vi "map_diag_piastre_stiffback.vi"() -> ()   [LabVIEW 2015]
panel:
  in  "x piastra":bool
  in  "y piastra":bool
  in  "z piastra":bool
  in  "Done":bool
  in  "y inizio":bool
  in  "Positioning Done":bool
  in  "x inizio":bool
  in  "y inizio":bool
  in  "Positioning Done":bool
  in  "y inizio":bool
  in  "Positioning Done":bool
  in  "KILL":bool
  in  "PAUSE":bool
  in  "RESUME":bool
  in  "QUIT":bool
  in  "Positioning Done":bool
  in  "y inizio":bool
  in  "x inizio":bool
  in  "End":bool
  in  "zero z - end":bool
  in  "zero x - end":bool
  in  "zero y - end":bool
  out "output":string
  out "command":string
  in  "zero done":bool
  in  "zero z":bool
  in  "zero x":bool
  in  "zero y":bool
  # "Posiziono in zero"
  # "Comandi di emergenza"
  # "Vado al punto di partenza\nDiagonale Left Internal"
  # "Vado al punto di partenza\nDiagonale Right Internal"
  # "Vado al punto di partenza\nDiagonale Left External"
  # "Vado al punto di partenza\nDiagonale Right External"
  # "Ritorno a zero"
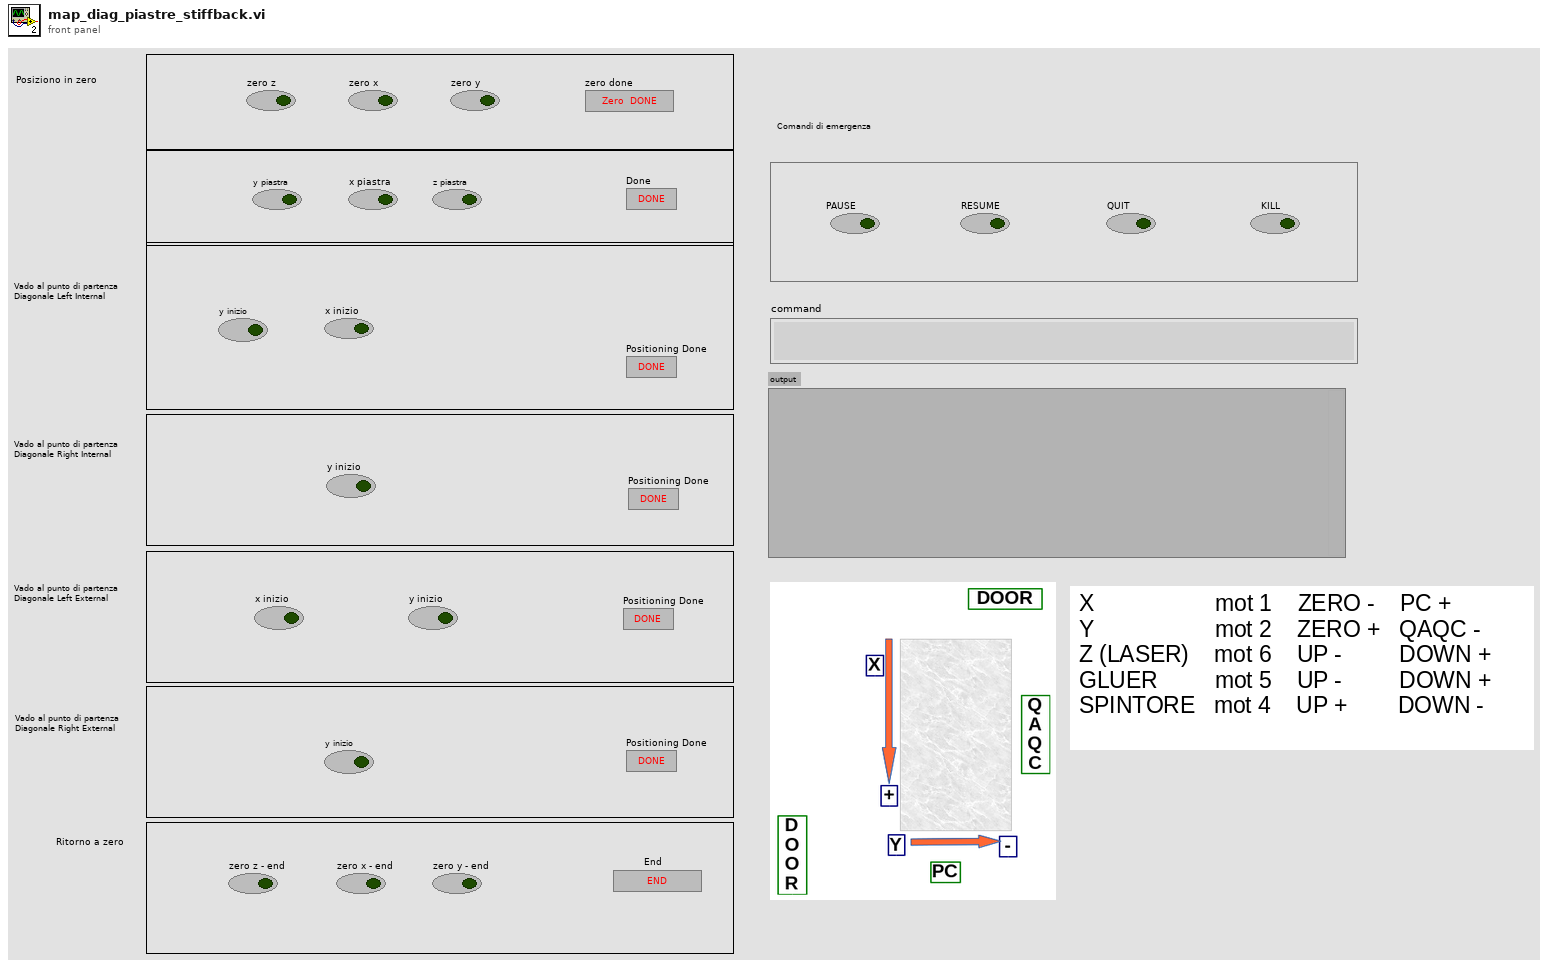
[diagram p1: front panel]
types:
  T1 = enum16{"open", "replace", "create", "open or create", "replace or create", "replace or create with confirmation"}
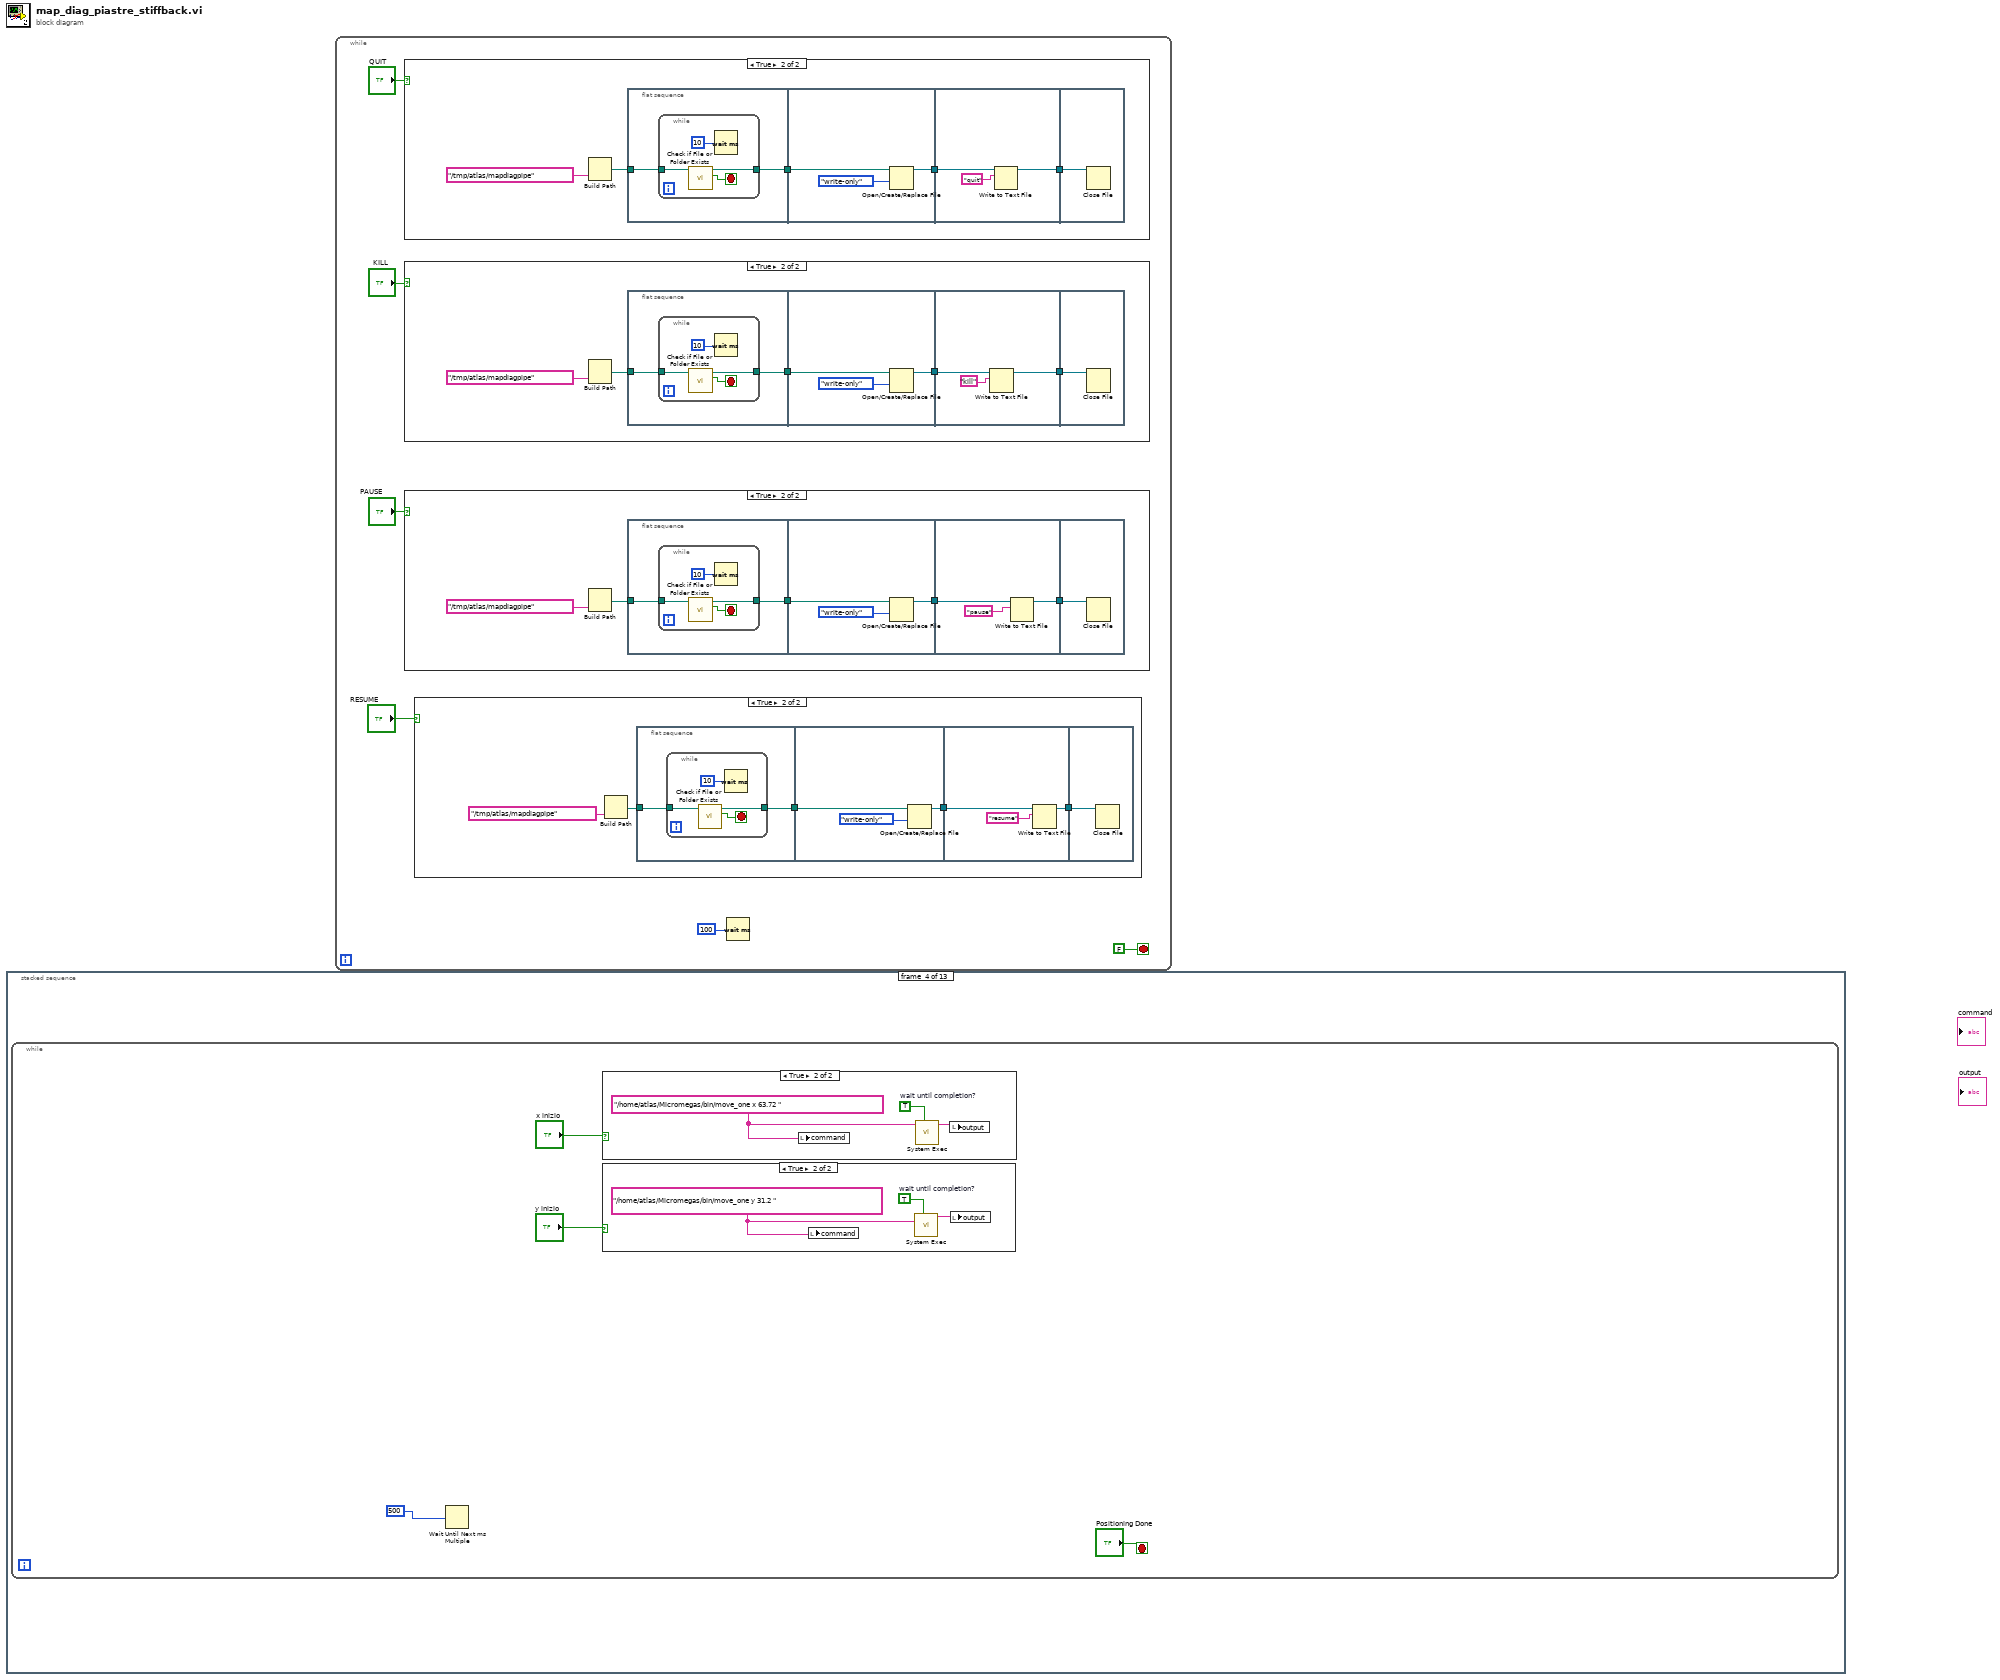
[diagram p0: block diagram]
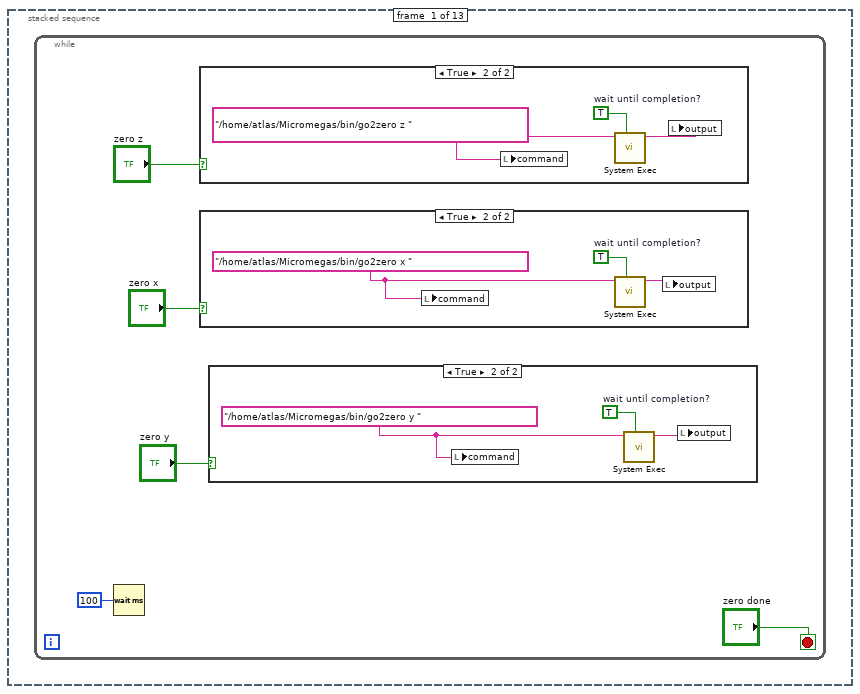
[diagram p6: hidden frame]
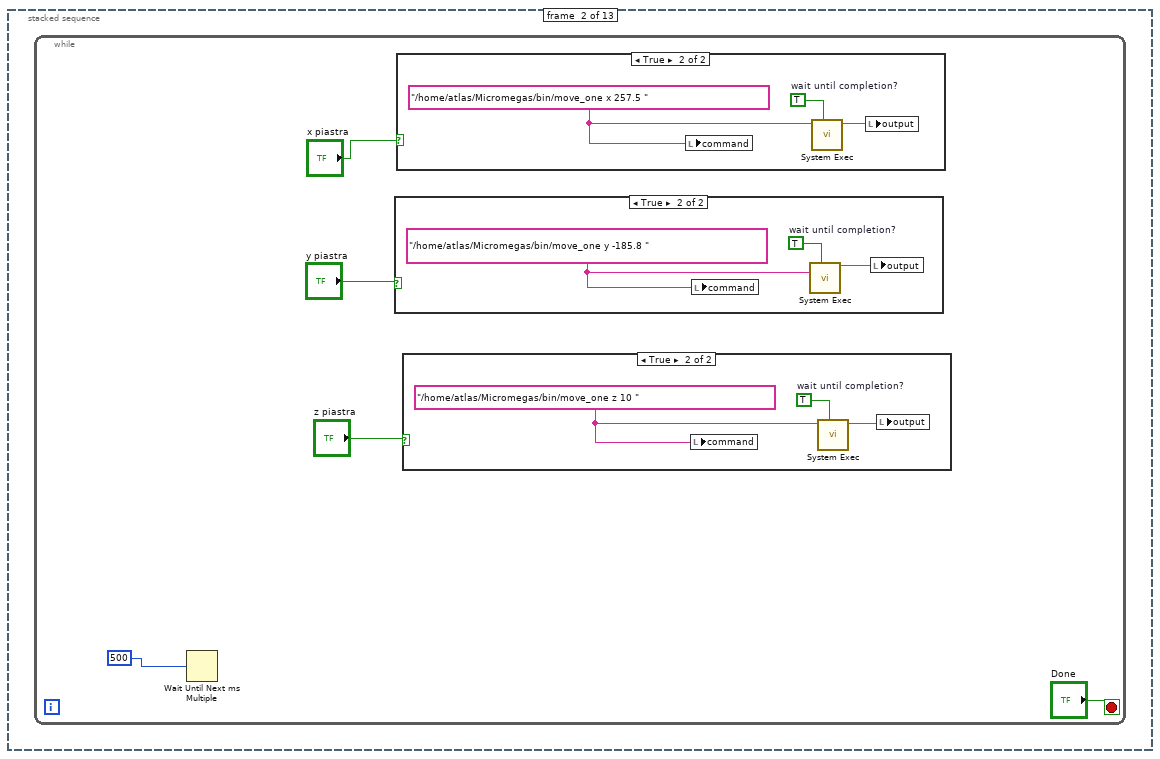
[diagram p10: hidden frame]
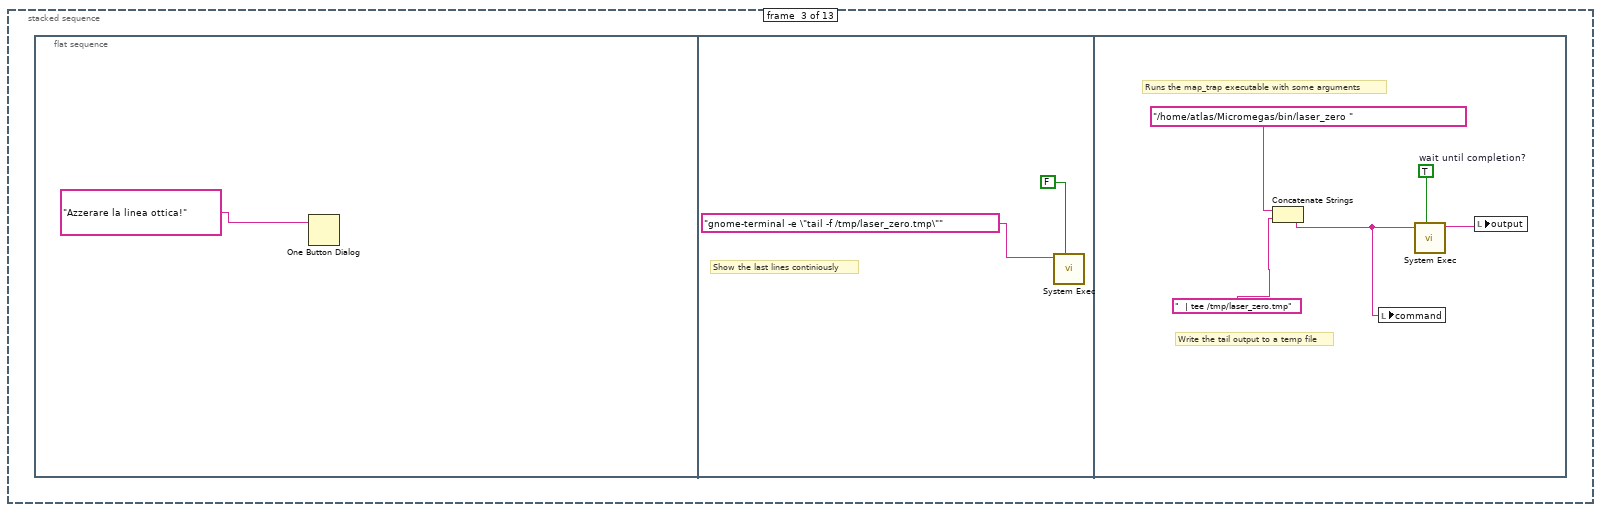
[diagram p14: hidden frame]
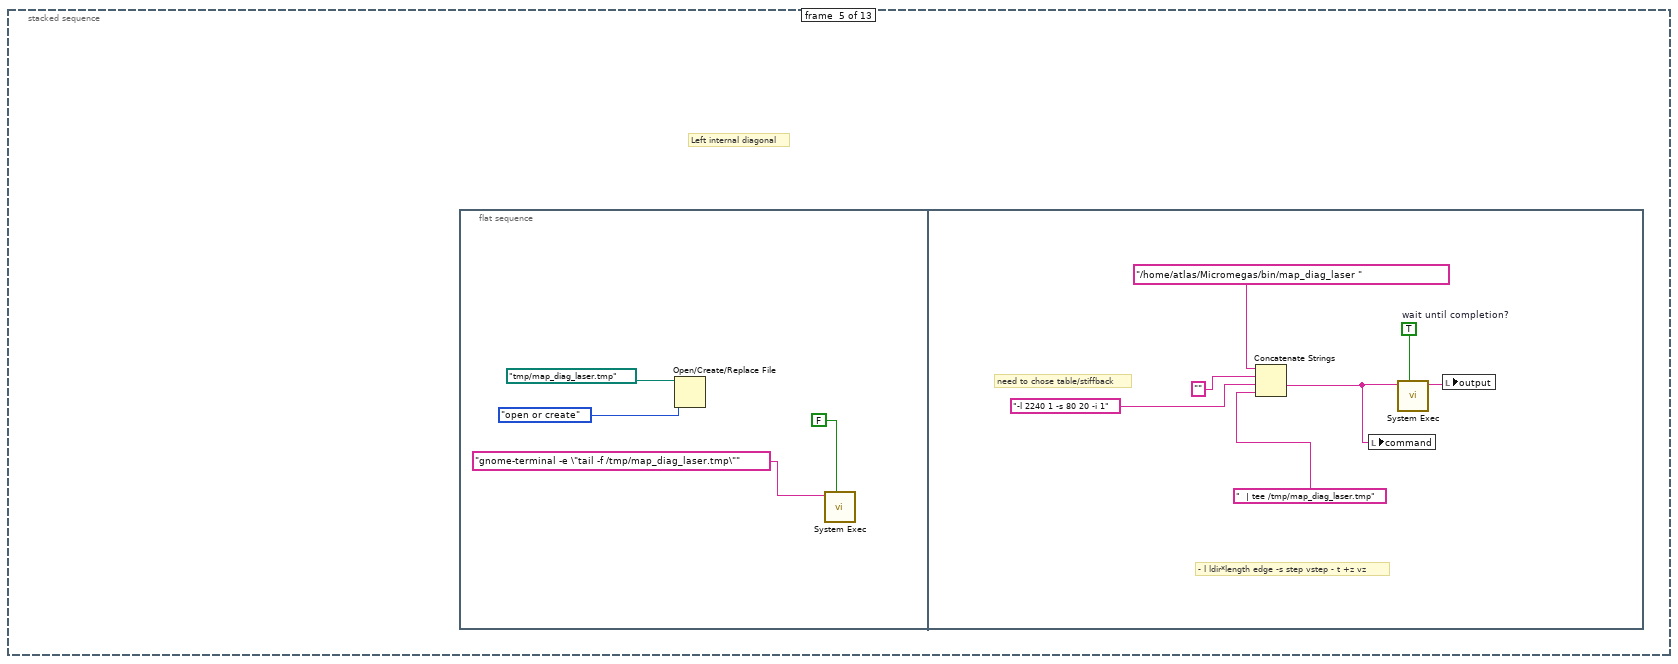
[diagram p17: hidden frame]
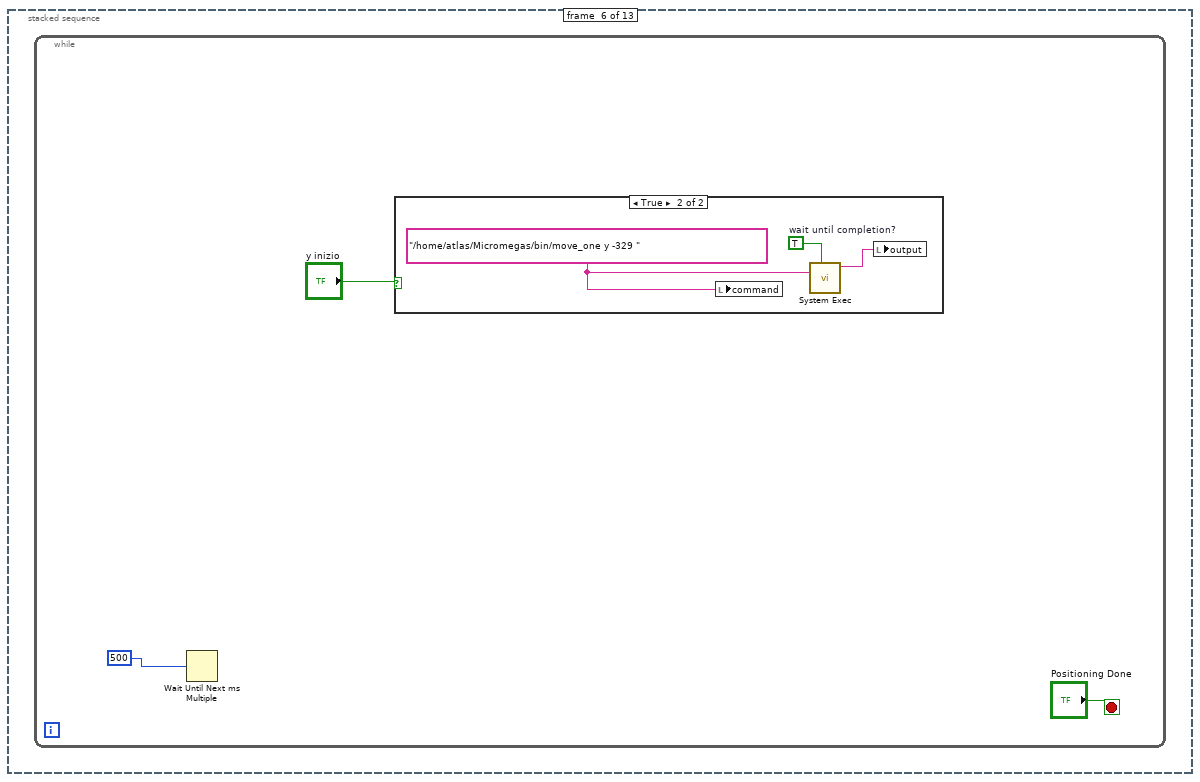
[diagram p18: hidden frame]
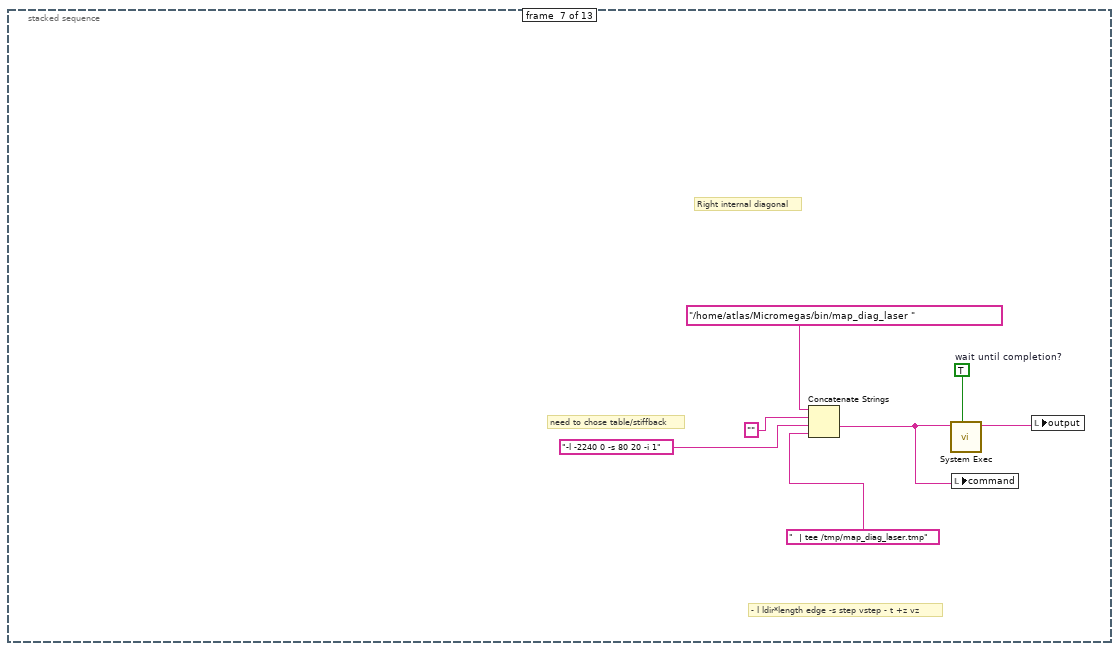
[diagram p20: hidden frame]
diagram:
  n1 = stacked-sequence {
    frame #0 {
      n2 = while {
        stop <- "zero done" stop-if-true
        n3 = Wait (ms)(milliseconds to wait=u32 100) -> ()  [unwired: 1 out]
        n4 = case shown="True" "zero z" {
          frame False {
          }
          frame True {
            w13 = "/home/atlas/Micromegas/bin/go2zero z " ("string")
            w14 = TRUE  # wait until completion?
            n5 = local write "command"(w13) -> ()
            n6 = call <vilib>:"System Exec.vi"("wait until completion? (T)"=w14, "command line"=w13) -> ("standard output"=w12:string)  [unwired: 6 in, 3 out]
            n7 = local write "output"(w12) -> ()
          }
        }
        n8 = case shown="True" "zero x" {
          frame False {
          }
          frame True {
            w10 = "/home/atlas/Micromegas/bin/go2zero x " ("string")
            w11 = TRUE  # wait until completion?
            n9 = local write "command"(w10) -> ()
            n10 = call <vilib>:"System Exec.vi"("wait until completion? (T)"=w11, "command line"=w10) -> ("standard output"=w9:string)  [unwired: 6 in, 3 out]
            n11 = local write "output"(w9) -> ()
          }
        }
        n12 = case shown="True" "zero y" {
          frame False {
          }
          frame True {
            w7 = "/home/atlas/Micromegas/bin/go2zero y " ("string")
            w8 = TRUE  # wait until completion?
            n13 = local write "command"(w7) -> ()
            n14 = call <vilib>:"System Exec.vi"("wait until completion? (T)"=w8, "command line"=w7) -> ("standard output"=w6:string)  [unwired: 6 in, 3 out]
            n15 = local write "output"(w6) -> ()
          }
        }
      }
    }
    frame #1 {
      n16 = while {
        stop <- "Done" stop-if-true
        n17 = Wait Until Next ms Multiple(millisecond multiple=u32 500 ("millisecond timer value")) -> ()  [unwired: 1 out]
        n18 = case shown="True" "y piastra" {
          frame False {
          }
          frame True {
            w23 = "/home/atlas/Micromegas/bin/move_one y -185.8 " ("string")
            w25 = TRUE  # wait until completion?
            n19 = local write "command"(w23) -> ()
            n20 = call <vilib>:"System Exec.vi"("wait until completion? (T)"=w25, "command line"=w23) -> ("standard output"=w24:string)  [unwired: 6 in, 3 out]
            n21 = local write "output"(w24) -> ()
          }
        }
        n22 = case shown="True" "x piastra" {
          frame False {
          }
          frame True {
            w26 = "/home/atlas/Micromegas/bin/move_one x 257.5 " ("string")
            w28 = TRUE  # wait until completion?
            n23 = local write "command"(w26) -> ()
            n24 = call <vilib>:"System Exec.vi"("wait until completion? (T)"=w28, "command line"=w26) -> ("standard output"=w27:string)  [unwired: 6 in, 3 out]
            n25 = local write "output"(w27) -> ()
          }
        }
        n26 = case shown="True" "z piastra" {
          frame False {
          }
          frame True {
            w21 = "/home/atlas/Micromegas/bin/move_one z 10 " ("string")
            w22 = TRUE  # wait until completion?
            n27 = local write "command"(w21) -> ()
            n28 = call <vilib>:"System Exec.vi"("wait until completion? (T)"=w22, "command line"=w21) -> ("standard output"=w20:string)  [unwired: 6 in, 3 out]
            n29 = local write "output"(w20) -> ()
          }
        }
      }
    }
    frame #2 {
      n30 = flat-sequence {
        frame #0 {
          n31 = One Button Dialog(message="Azzerare la linea ottica!") -> ()  [unwired: 1 in, 1 out]
        }
        frame #1 {
          # "Show the last lines continiously"
          n32 = call <vilib>:"System Exec.vi"("wait until completion? (T)"=FALSE, "command line"="gnome-terminal -e \"tail -f /tmp/laser_zero.tmp\"") -> ()  [unwired: 6 in, 4 out]
        }
        frame #2 {
          w36 = TRUE  # wait until completion?
          # "Write the tail output to a temp file"
          # "Runs the map_trap executable with some arguments"
          n33 = Concatenate Strings("/home/atlas/Micromegas/bin/laser_zero " ("string"), "  | tee /tmp/laser_zero.tmp" ("string")) -> (w32:string)
          n34 = local write "command"(w32) -> ()
          n35 = call <vilib>:"System Exec.vi"("wait until completion? (T)"=w36, "command line"=w32) -> ("standard output"=w33:string)  [unwired: 6 in, 3 out]
          n36 = local write "output"(w33) -> ()
        }
      }
    }
    frame #3 {
      n37 = while {
        stop <- "Positioning Done" stop-if-true
        n38 = Wait Until Next ms Multiple(millisecond multiple=u32 500 ("millisecond timer value")) -> ()  [unwired: 1 out]
        n39 = case shown="True" "y inizio" {
          frame False {
          }
          frame True {
            w41 = "/home/atlas/Micromegas/bin/move_one y 31.2 " ("string")
            w43 = TRUE  # wait until completion?
            n40 = local write "command"(w41) -> ()
            n41 = call <vilib>:"System Exec.vi"("wait until completion? (T)"=w43, "command line"=w41) -> ("standard output"=w42:string)  [unwired: 6 in, 3 out]
            n42 = local write "output"(w42) -> ()
          }
        }
        n43 = case shown="True" "x inizio" {
          frame False {
          }
          frame True {
            w44 = "/home/atlas/Micromegas/bin/move_one x 63.72 " ("string")
            w46 = TRUE  # wait until completion?
            n44 = local write "command"(w44) -> ()
            n45 = call <vilib>:"System Exec.vi"("wait until completion? (T)"=w46, "command line"=w44) -> ("standard output"=w45:string)  [unwired: 6 in, 3 out]
            n46 = local write "output"(w45) -> ()
          }
        }
      }
    }
    frame #4 {
      # "Left internal diagonal"
      n47 = flat-sequence {
        frame #0 {
          n48 = Open/Create/Replace File(file path (use dialog)=path "/tmp/map_diag_laser.tmp", operation (0:open)=T1."open or create") -> ()  [unwired: 4 in, 3 out]
          n49 = call <vilib>:"System Exec.vi"("wait until completion? (T)"=FALSE, "command line"="gnome-terminal -e \"tail -f /tmp/map_diag_laser.tmp\"") -> ()  [unwired: 6 in, 4 out]
        }
        frame #1 {
          w57 = TRUE  # wait until completion?
          # "need to chose table/stiffback"
          # "- l ldir*length edge -s step vstep - t +z vz"
          n50 = Concatenate Strings("/home/atlas/Micromegas/bin/map_diag_laser " ("string"), "" ("string"), "-l 2240 1 -s 80 20 -i 1" ("string"), "  | tee /tmp/map_diag_laser.tmp" ("string")) -> (w54:string)
          n51 = local write "command"(w54) -> ()
          n52 = call <vilib>:"System Exec.vi"("wait until completion? (T)"=w57, "command line"=w54) -> ("standard output"=w55:string)  [unwired: 6 in, 3 out]
          n53 = local write "output"(w55) -> ()
        }
      }
    }
    frame #5 {
      n54 = while {
        stop <- "Positioning Done" stop-if-true
        n55 = Wait Until Next ms Multiple(millisecond multiple=u32 500 ("millisecond timer value")) -> ()  [unwired: 1 out]
        n56 = case shown="True" "y inizio" {
          frame False {
          }
          frame True {
            w61 = "/home/atlas/Micromegas/bin/move_one y -329 " ("string")
            w63 = TRUE  # wait until completion?
            n57 = local write "command"(w61) -> ()
            n58 = call <vilib>:"System Exec.vi"("wait until completion? (T)"=w63, "command line"=w61) -> ("standard output"=w62:string)  [unwired: 6 in, 3 out]
            n59 = local write "output"(w62) -> ()
          }
        }
      }
    }
    frame #6 {
      w70 = TRUE  # wait until completion?
      # "Right internal diagonal"
      # "need to chose table/stiffback"
      # "- l ldir*length edge -s step vstep - t +z vz"
      n60 = Concatenate Strings("/home/atlas/Micromegas/bin/map_diag_laser " ("string"), "" ("string"), "-l -2240 0 -s 80 20 -i 1" ("string"), "  | tee /tmp/map_diag_laser.tmp" ("string")) -> (w64:string)
      n61 = call <vilib>:"System Exec.vi"("wait until completion? (T)"=w70, "command line"=w64) -> ("standard output"=w65:string)  [unwired: 6 in, 3 out]
      n62 = local write "command"(w64) -> ()
      n63 = local write "output"(w65) -> ()
    }
    frame #7 {
      n64 = while {
        stop <- "Positioning Done" stop-if-true
        n65 = Wait Until Next ms Multiple(millisecond multiple=u32 500 ("millisecond timer value")) -> ()  [unwired: 1 out]
        n66 = case shown="True" "x inizio" {
          frame False {
          }
          frame True {
            w75 = "/home/atlas/Micromegas/bin/move_one x 11 " ("string")
            w77 = TRUE  # wait until completion?
            n67 = local write "command"(w75) -> ()
            n68 = call <vilib>:"System Exec.vi"("wait until completion? (T)"=w77, "command line"=w75) -> ("standard output"=w76:string)  [unwired: 6 in, 3 out]
            n69 = local write "output"(w76) -> ()
          }
        }
        n70 = case shown="True" "y inizio" {
          frame False {
          }
          frame True {
            w78 = "/home/atlas/Micromegas/bin/move_one y 1190 " ("string")
            w80 = TRUE  # wait until completion?
            n71 = local write "command"(w78) -> ()
            n72 = call <vilib>:"System Exec.vi"("wait until completion? (T)"=w80, "command line"=w78) -> ("standard output"=w79:string)  [unwired: 6 in, 3 out]
            n73 = local write "output"(w79) -> ()
          }
        }
      }
    }
    frame #8 {
      w87 = TRUE  # wait until completion?
      # "Left external diagonal"
      # "need to chose table/stiffback"
      # "- l ldir*length edge -s step vstep - t +z vz"
      n74 = Concatenate Strings("/home/atlas/Micromegas/bin/map_diag_laser " ("string"), "" ("string"), "-l 2200 1 -s 110 20 -i 1" ("string"), "  | tee /tmp/map_diag_laser.tmp" ("string")) -> (w81:string)
      n75 = call <vilib>:"System Exec.vi"("wait until completion? (T)"=w87, "command line"=w81) -> ("standard output"=w82:string)  [unwired: 6 in, 3 out]
      n76 = local write "command"(w81) -> ()
      n77 = local write "output"(w82) -> ()
    }
    frame #9 {
      n78 = while {
        stop <- "Positioning Done" stop-if-true
        n79 = Wait Until Next ms Multiple(millisecond multiple=u32 500 ("millisecond timer value")) -> ()  [unwired: 1 out]
        n80 = case shown="True" "y inizio" {
          frame False {
          }
          frame True {
            w91 = "/home/atlas/Micromegas/bin/move_one y -505 " ("string")
            w93 = TRUE  # wait until completion?
            n81 = local write "command"(w91) -> ()
            n82 = call <vilib>:"System Exec.vi"("wait until completion? (T)"=w93, "command line"=w91) -> ("standard output"=w92:string)  [unwired: 6 in, 3 out]
            n83 = local write "output"(w92) -> ()
          }
        }
      }
    }
    frame #10 {
      w100 = TRUE  # wait until completion?
      # "Right external diagonal"
      # "need to chose table/stiffback"
      # "- l ldir*length edge -s step vstep - t +z vz"
      n84 = Concatenate Strings("/home/atlas/Micromegas/bin/map_diag_laser " ("string"), "" ("string"), "-l -2200 0 -s 110 20 -i 1" ("string"), "  | tee /tmp/map_diag_laser.tmp" ("string")) -> (w94:string)
      n85 = call <vilib>:"System Exec.vi"("wait until completion? (T)"=w100, "command line"=w94) -> ("standard output"=w95:string)  [unwired: 6 in, 3 out]
      n86 = local write "command"(w94) -> ()
      n87 = local write "output"(w95) -> ()
    }
    frame #11 {
      n88 = while {
        stop <- "End" stop-if-true
        n89 = Wait (ms)(milliseconds to wait=u32 100) -> ()  [unwired: 1 out]
        n90 = case shown="True" "zero z - end" {
          frame False {
          }
          frame True {
            w113 = "/home/atlas/Micromegas/bin/go2zero z " ("string")
            w114 = TRUE  # wait until completion?
            n91 = local write "command"(w113) -> ()
            n92 = call <vilib>:"System Exec.vi"("wait until completion? (T)"=w114, "command line"=w113) -> ("standard output"=w112:string)  [unwired: 6 in, 3 out]
            n93 = local write "output"(w112) -> ()
          }
        }
        n94 = case shown="True" "zero x - end" {
          frame False {
          }
          frame True {
            w110 = "/home/atlas/Micromegas/bin/go2zero x " ("string")
            w111 = TRUE  # wait until completion?
            n95 = local write "command"(w110) -> ()
            n96 = call <vilib>:"System Exec.vi"("wait until completion? (T)"=w111, "command line"=w110) -> ("standard output"=w109:string)  [unwired: 6 in, 3 out]
            n97 = local write "output"(w109) -> ()
          }
        }
        n98 = case shown="True" "zero y - end" {
          frame False {
          }
          frame True {
            w107 = "/home/atlas/Micromegas/bin/go2zero y " ("string")
            w108 = TRUE  # wait until completion?
            n99 = local write "command"(w107) -> ()
            n100 = call <vilib>:"System Exec.vi"("wait until completion? (T)"=w108, "command line"=w107) -> ("standard output"=w106:string)  [unwired: 6 in, 3 out]
            n101 = local write "output"(w106) -> ()
          }
        }
      }
    }
    frame #12 {
      n102 = One Button Dialog(message="Per comodita`, rinominare il file (non verra` comunque sovrascritto)") -> ()  [unwired: 1 in, 1 out]
    }
  }
  n103 = while {
    stop <- FALSE stop-if-true
    n104 = case shown="True" "QUIT" {
      frame False {
      }
      frame True {
        n105 = Build Path(name or relative path="/tmp/atlas/mapdiagpipe" ("string")) -> (appended path=w176:path)  [unwired: 1 in]
        n106 = flat-sequence {
          tunnel: [w182] -> w180
          tunnel: w176 -> [w181]
          tunnel: w180 -> [w189]
          tunnel: [w187] -> w179
          tunnel: w179 -> [w192]
          tunnel: [w191] -> w178
          tunnel: w178 -> [w193]
          frame #0 {
            n107 = while {
              tunnel: [w184] -> w182
              tunnel: w181 -> [w183]
              stop <- w185 stop-if-true
              n108 = call <vilib>:"Check if File or Folder Exists.vi"("path"=w183) -> ("file or folder exists?"=w185:bool, "dup path"=w184:path)  [unwired: 8 in, 1 out]
              n109 = Wait (ms)(milliseconds to wait=u32 10) -> ()  [unwired: 1 out]
            }
          }
          frame #1 {
            n110 = Open/Create/Replace File(file path (use dialog)=w189, access (0:read/write)=enum16{"read/write", "read-only", "write-only"}."write-only") -> (refnum out=w187:refnum<file>)  [unwired: 4 in, 2 out]
          }
          frame #2 {
            n111 = Write to Text File(file (use dialog)=w192, text="quit") -> (refnum out=w191:refnum<file>)  [unwired: 2 in, 2 out]
          }
          frame #3 {
            n112 = Close File(refnum=w193) -> ()  [unwired: 1 in, 2 out]
          }
        }
      }
    }
    n113 = case shown="True" "KILL" {
      frame False {
      }
      frame True {
        n114 = Build Path(name or relative path="/tmp/atlas/mapdiagpipe" ("string")) -> (appended path=w140:path)  [unwired: 1 in]
        n115 = flat-sequence {
          tunnel: [w146] -> w144
          tunnel: w140 -> [w145]
          tunnel: w144 -> [w153]
          tunnel: [w151] -> w143
          tunnel: w143 -> [w156]
          tunnel: [w155] -> w142
          tunnel: w142 -> [w157]
          frame #0 {
            n116 = while {
              tunnel: [w148] -> w146
              tunnel: w145 -> [w147]
              stop <- w149 stop-if-true
              n117 = call <vilib>:"Check if File or Folder Exists.vi"("path"=w147) -> ("file or folder exists?"=w149:bool, "dup path"=w148:path)  [unwired: 8 in, 1 out]
              n118 = Wait (ms)(milliseconds to wait=u32 10) -> ()  [unwired: 1 out]
            }
          }
          frame #1 {
            n119 = Open/Create/Replace File(file path (use dialog)=w153, access (0:read/write)=enum16{"read/write", "read-only", "write-only"}."write-only") -> (refnum out=w151:refnum<file>)  [unwired: 4 in, 2 out]
          }
          frame #2 {
            n120 = Write to Text File(file (use dialog)=w156, text="kill") -> (refnum out=w155:refnum<file>)  [unwired: 2 in, 2 out]
          }
          frame #3 {
            n121 = Close File(refnum=w157) -> ()  [unwired: 1 in, 2 out]
          }
        }
      }
    }
    n122 = case shown="True" "PAUSE" {
      frame False {
      }
      frame True {
        n123 = Build Path(name or relative path="/tmp/atlas/mapdiagpipe" ("string")) -> (appended path=w122:path)  [unwired: 1 in]
        n124 = flat-sequence {
          tunnel: [w128] -> w126
          tunnel: w122 -> [w127]
          tunnel: w126 -> [w135]
          tunnel: [w133] -> w125
          tunnel: w125 -> [w138]
          tunnel: [w137] -> w124
          tunnel: w124 -> [w139]
          frame #0 {
            n125 = while {
              tunnel: [w130] -> w128
              tunnel: w127 -> [w129]
              stop <- w131 stop-if-true
              n126 = call <vilib>:"Check if File or Folder Exists.vi"("path"=w129) -> ("file or folder exists?"=w131:bool, "dup path"=w130:path)  [unwired: 8 in, 1 out]
              n127 = Wait (ms)(milliseconds to wait=u32 10) -> ()  [unwired: 1 out]
            }
          }
          frame #1 {
            n128 = Open/Create/Replace File(file path (use dialog)=w135, access (0:read/write)=enum16{"read/write", "read-only", "write-only"}."write-only") -> (refnum out=w133:refnum<file>)  [unwired: 4 in, 2 out]
          }
          frame #2 {
            n129 = Write to Text File(file (use dialog)=w138, text="pause") -> (refnum out=w137:refnum<file>)  [unwired: 2 in, 2 out]
          }
          frame #3 {
            n130 = Close File(refnum=w139) -> ()  [unwired: 1 in, 2 out]
          }
        }
      }
    }
    n131 = case shown="True" "RESUME" {
      frame False {
      }
      frame True {
        n132 = Build Path(name or relative path="/tmp/atlas/mapdiagpipe" ("string")) -> (appended path=w158:path)  [unwired: 1 in]
        n133 = flat-sequence {
          tunnel: [w164] -> w162
          tunnel: w158 -> [w163]
          tunnel: w162 -> [w171]
          tunnel: [w169] -> w161
          tunnel: w161 -> [w174]
          tunnel: [w173] -> w160
          tunnel: w160 -> [w175]
          frame #0 {
            n134 = while {
              tunnel: [w166] -> w164
              tunnel: w163 -> [w165]
              stop <- w167 stop-if-true
              n135 = call <vilib>:"Check if File or Folder Exists.vi"("path"=w165) -> ("file or folder exists?"=w167:bool, "dup path"=w166:path)  [unwired: 8 in, 1 out]
              n136 = Wait (ms)(milliseconds to wait=u32 10) -> ()  [unwired: 1 out]
            }
          }
          frame #1 {
            n137 = Open/Create/Replace File(file path (use dialog)=w171, access (0:read/write)=enum16{"read/write", "read-only", "write-only"}."write-only") -> (refnum out=w169:refnum<file>)  [unwired: 4 in, 2 out]
          }
          frame #2 {
            n138 = Write to Text File(file (use dialog)=w174, text="resume") -> (refnum out=w173:refnum<file>)  [unwired: 2 in, 2 out]
          }
          frame #3 {
            n139 = Close File(refnum=w175) -> ()  [unwired: 1 in, 2 out]
          }
        }
      }
    }
    n140 = Wait (ms)(milliseconds to wait=100) -> ()  [unwired: 1 out]
  }
